vi "FPGA_controller.vi"() -> ()   [LabVIEW 2017]
uses:
  <vilib>/rvi/Emulation/niFpgaGetClockAttributes.vi
  <vilib>/rvi/Emulation/niFpgaSctlEmulationGetInTimedLoop.vi
  <vilib>/rvi/Emulation/niFpgaEmulationReportErrorSimple.vi
  <vilib>/rvi/eio/common/nirviEmuTemplateMethod_errors.vi
  <vilib>/rvi/Emulation/niFpgaCriticalErrorInLSC.vi
  <vilib>/eio/EIONode/EIONode.xnode
panel:
  in  "Scale x2":fxp<+/-,32,16>=10.0 format="%#_21g"
  in  "m_first x2":fxp<+/-,49,33>=4.9499969482421875 format="%#_26g"
  in  "Offset x2":fxp<+/-,48,32> format="%#_26g"
  in  "1/eta x":fxp<+,8,8>=200.0 format="%#_21g"
  in  "m_first x1":fxp<+/-,49,33>=0.649993896484375 format="%#_26g"
  in  "Offset x1":fxp<+/-,48,32> format="%#_26g"
  in  "Scale x1":fxp<+/-,32,16>=5.0 format="%#_21g"
  in  "stop 2":bool
  # "STATES CONVERSION"
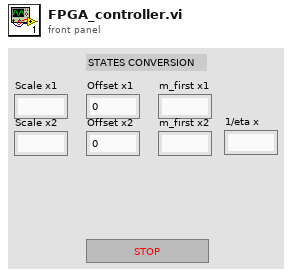
[diagram p1: front panel]
types:
  T1 = cluster{"Boolean array[0]":bool, "Boolean array[1]":bool, "Boolean array[2]":bool, "Boolean array[3]":bool, "Boolean array[4]":bool, "Boolean array[5]":bool, "Boolean array[6]":bool, "Boolean array[7]":bool, "Boolean array[8]":bool, "Boolean array[9]":bool, "Boolean array[10]":bool, "Boolean array[11]":bool, "Boolean array[12]":bool, "Boolean array[13]":bool, "Boolean array[14]":bool, "Boolean array[15]":bool}
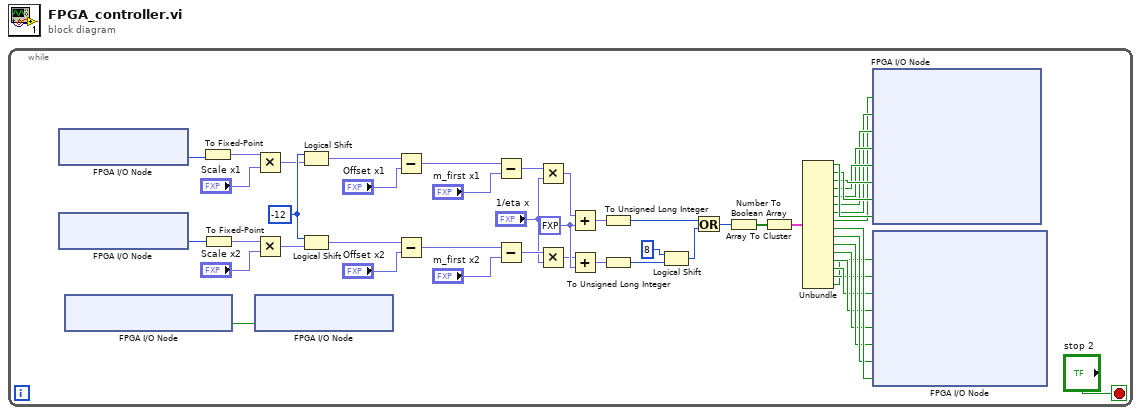
[diagram p0: block diagram]
diagram:
  n1 = while {
    stop <- "stop 2" stop-if-true
    w26 = fxp<+,2,1> 0.5 ("y")
    w24 = i16 -12 ("y")
    n2 = xnode "FPGA I/O Node"() -> ("ConnectorA/AI0"=w4:u16)  [unwired: 1 in, 1 out]
    n3 = xnode "FPGA I/O Node"() -> ("ConnectorA/AI1"=w2:u16)  [unwired: 1 in, 1 out]
    n4 = xnode "FPGA I/O Node"() -> ("Component-Level IP\\f0"=w33:bool)  [unwired: 1 in, 1 out]
    n5 = To Fixed-Point(number=w4) -> (fixed-point=w3:fxp<+,16,16>)  [unwired: 1 in]
    n6 = To Fixed-Point(number=w2) -> (fixed-point=w1:fxp<+,16,16>)  [unwired: 1 in]
    n7 = Multiply(x=w3, y="Scale x1") -> (x*y=w23:fxp<+/-,48,32>)
    n8 = Multiply(x=w1, y="Scale x2") -> (x*y=w27:fxp<+/-,48,32>)
    n9 = xnode "FPGA I/O Node"("ConnectorA/DIO0"=w33) -> ()  [unwired: 1 in, 1 out]
    n10 = Logical Shift(y=w24, x=w23) -> (x << y=w20:fxp<+/-,48,32>)
    n11 = Logical Shift(y=w24, x=w27) -> (x << y=w17:fxp<+/-,48,32>)
    n12 = Subtract(x=w20, y="Offset x1") -> (x-y=w21:fxp<+/-,49,33>)
    n13 = Subtract(x=w17, y="Offset x2") -> (x-y=w18:fxp<+/-,49,33>)
    n14 = Subtract(x=w21, y="m_first x1") -> (x-y=w22:fxp<+/-,50,34>)
    n15 = Subtract(x=w18, y="m_first x2") -> (x-y=w16:fxp<+/-,50,34>)
    n16 = Multiply(x=w22, y="1/eta x") -> (x*y=w19:fxp<+/-,58,42>)
    n17 = Multiply(x=w16, y="1/eta x") -> (x*y=w15:fxp<+/-,58,42>)
    n18 = Add(x=w19, y=w26) -> (x+y=w32:fxp<+/-,58,42>)
    n19 = Add(x=w15, y=w26) -> (x+y=w25:fxp<+/-,58,42>)
    n20 = To Unsigned Long Integer(number=w32) -> (unsigned 32bit integer=w28:u32)
    n21 = To Unsigned Long Integer(number=w25) -> (unsigned 32bit integer=w30:u32)
    n22 = Logical Shift(y=8, x=w30) -> (x << y=w29:u32)
    n23 = Or(x=w28, y=w29) -> (x .or. y?=w12:u32)
    n24 = Number To Boolean Array(number=w12) -> (Boolean array=w13:bool[])
    n25 = Array To Cluster(array=w13) -> (cluster=w50:T1)
    n26 = Unbundle(w50) -> ("Boolean array[0]"=w49:bool, "Boolean array[1]"=w48:bool, "Boolean array[2]"=w47:bool, "Boolean array[3]"=w46:bool, "Boolean array[4]"=w45:bool, "Boolean array[5]"=w44:bool, "Boolean array[6]"=w43:bool, "Boolean array[7]"=w42:bool, "Boolean array[8]"=w41:bool, "Boolean array[9]"=w40:bool, "Boolean array[10]"=w39:bool, "Boolean array[11]"=w38:bool, "Boolean array[12]"=w37:bool, "Boolean array[13]"=w36:bool, "Boolean array[14]"=w35:bool, "Boolean array[15]"=w34:bool)
    n27 = xnode "FPGA I/O Node"("Component-Level IP\\x0"=w42, "Component-Level IP\\x1"=w43, "Component-Level IP\\x2"=w44, "Component-Level IP\\x3"=w45, "Component-Level IP\\x4"=w46, "Component-Level IP\\x5"=w47, "Component-Level IP\\x6"=w48, "Component-Level IP\\x7"=w49) -> ()  [unwired: 8 in, 8 out]
    n28 = xnode "FPGA I/O Node"("Component-Level IP\\x8"=w34, "Component-Level IP\\x9"=w35, "Component-Level IP\\x10"=w36, "Component-Level IP\\x11"=w37, "Component-Level IP\\x12"=w38, "Component-Level IP\\x13"=w39, "Component-Level IP\\x14"=w40, "Component-Level IP\\x15"=w41) -> ()  [unwired: 8 in, 8 out]
  }
